vi "Wait For Session Status.vi"(7 "Timeout (3000 ms)":u32=3000, 8 "error in (no error)":errorcluster, 10 "IN_SESSION State (T)":bool=TRUE, 11 "VISA Resource Name":refnum<visa-resource-name>) -> (0 "error out":errorcluster, 1 "Elapsed Time (ms)":u32, 2 "IN_SESSION":bool, 3 "dup VISA Resource Name":refnum<visa-resource-name>)   [LabVIEW 2020]
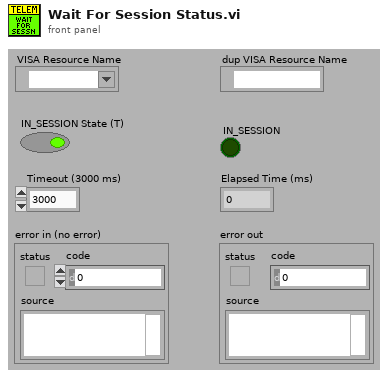
[diagram p1: front panel]
types:
  T1 = cluster{"ERROR_OCCURRED":bool, "LINK_STAT_CHANGED":bool, "LINK_QUAL_CHANGED":bool, "400MHZ_TX_ACTIVE":bool, "400MHZ_RX_ACTIVE":bool, "245GHZ_TX_ACTIVE":bool, "DATA_STAT_CHANGED":bool, "SLEEPING":bool, "IDLE":bool, "SEARCHING_FOR_IMPLANT":bool, "STARTING_SESSION":bool, "LISTENING_FOR_EMERG":bool, "IN_SESSION":bool}
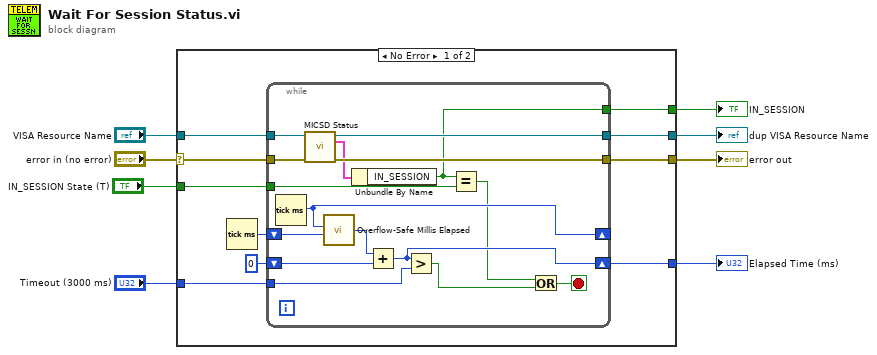
[diagram p0: block diagram]
diagram:
  n1 = case shown="No Error" "error in (no error)" {
    selector: "error in (no error)" -> [w11 w36]
    tunnel: [w18 _] -> w8
    tunnel: "VISA Resource Name" -> [w15 w35]
    tunnel: [w14 _] -> w6
    tunnel: [w13 w35] -> w5
    tunnel: [w12 w36] -> w4
    tunnel: "Timeout (3000 ms)" -> [w10 _]
    tunnel: "IN_SESSION State (T)" -> [w9 _]
    frame No Error {
      n2 = Tick Count (ms)() -> (millisecond timer value=w16:u32)
      n3 = while {
        tunnel: [w34] -> w12
        tunnel: [w33] -> w13
        shift-right: [w26] -> _
        shift-left: w16 -> [w31]
        tunnel: [w20] -> w14
        tunnel: w11 -> [w28]
        tunnel: w15 -> [w27]
        shift-right: [w23] -> w18
        shift-left: u32 0 ("millisecond timer value") -> [w25]
        tunnel: w10 -> [w22]
        tunnel: w9 -> [w21]
        stop <- w29 stop-if-true
        n4 = Tick Count (ms)() -> (millisecond timer value=w26:u32)
        n5 = call "MICSD Status.vi"("VISA Resource Name"=w27, "error in (no error)"=w28) -> ("dup VISA Resource Name"=w33:refnum<visa-resource-name>, "Status Flags"=w30:T1, "error out"=w34:errorcluster)  [unwired: 7 in, 4 out]
        n6 = call "Overflow-Safe Millis Elapsed.vi"("now"=w26, "previous"=w31) -> ("elapsed"=w24:u32)  [unwired: 5 in]
        n7 = Unbundle By Name(w30) -> ("IN_SESSION"=w20:bool)
        n8 = Add(x=w24, y=w25) -> (x+y=w23:u32)
        n9 = Greater?(x=w23, y=w22) -> (0:w32:bool)
        n10 = Equal?(x=w20, y=w21) -> (x = y?=w19:bool)
        n11 = Or(x=w19, y=w32) -> (x .or. y?=w29:bool)
      }
    }
    frame Error {
    }
  }
  "Elapsed Time (ms)" <- w8
  "IN_SESSION" <- w6
  "dup VISA Resource Name" <- w5
  "error out" <- w4
